vi "FF_TInial_pel.vi"() -> (0 "xyz_o":dbl[][](array[numeric]), 3 "Array":T1[](array[typedef]))   [LabVIEW 2017]
uses:
  typeDef/AnkleTraj.ctl
  <vilib>/Analysis/baseanly.llb/Real Dot Product.vi
  <vilib>/imath/engines/lvmath2/RunTimeEngine/Managers/WorkSpace/UID Generator.vi
  <vilib>/imath/engines/lvmath2/RunTimeEngine/RunTimeType/NIMS_RunTimeType_From StrictType (excl LVString).vi
  <instcachedir>/0/NIMS_RunTimeType_From StrictType (excl LVString)_1019F277F0A747EDBCA0F6C52CA54500.lvgen/NIMS_RunTimeType_From StrictType (excl LVString)_1019F277F0A747EDBCA0F6C52CA54500_000.vi
  <vilib>/imath/engines/lvmath2/RunTimeEngine/LocalVariableDefStatement/MC_LocalVariableDefStatement_Display.vi
  <vilib>/imath/engines/lvmath2/RunTimeEngine/RangeToken/NIMS_Range_R2 - Integer.vi
  <instcachedir>/0/NIMS_Range_R2 - Integer_B2C3C6B11D0E4F789E1772ACB483EB02.lvgen/NIMS_Range_R2 - Integer_B2C3C6B11D0E4F789E1772ACB483EB02_000.vi
  <vilib>/imath/engines/lvmath2/RunTimeEngine/CommandStatement/MC_CommandStatement_break.vi
  <vilib>/imath/engines/lvmath2/RunTimeEngine/VariableToken/NIMS_VariableToken_CondDefinedDefinedByReplace.vi
  <instcachedir>/0/NIMS_VariableToken_CondDefinedDefinedByReplace_D162CFFC24174562A9FEA619A91E1A56.lvgen/NIMS_VariableToken_CondDefinedDefinedByReplace_D162CFFC24174562A9FEA619A91E1A56_002.vi
  <vilib>/imath/engines/lvmath2/RunTimeEngine/IndexReplace/NIMS V(S)=S.vi
  <instcachedir>/0/NIMS V(S)=S_3F4D177D41884A9C969E5FA0B22E4B28.lvgen/NIMS V(S)=S_3F4D177D41884A9C969E5FA0B22E4B28_000.vi
  <vilib>/imathl/engines/lvmath/Functions/Error Handling/Create Error.vi
  <vilib>/imath/engines/lvmath2/RunTimeEngine/VariableToken/NIMS_VariableToken_CondDefined.vi
  <instcachedir>/0/NIMS_VariableToken_CondDefined_6E7F1EE7F80E48298C84CF05BD736261.lvgen/NIMS_VariableToken_CondDefined_6E7F1EE7F80E48298C84CF05BD736261_003.vi
  <vilib>/imath/engines/lvmath2/RunTimeEngine/BuiltInFunctions/transpose/NIMS_transpose(GV).vi
  <instcachedir>/0/NIMS_transpose(GV)_1D76875BF542458FA31D2D0CC3E998C0.lvgen/NIMS_transpose(GV)_1D76875BF542458FA31D2D0CC3E998C0_000.vi
  <vilib>/imath/engines/lvmath2/RunTimeEngine/IndexReplace/NIMS M($,S)=V.vi
  <instcachedir>/0/NIMS M($,S)=V_A7D5EE67177749758173A2B7AA759022.lvgen/NIMS M($,S)=V_A7D5EE67177749758173A2B7AA759022_001.vi
  <vilib>/imath/engines/lvmath2/RunTimeEngine/ErrorHandling/NIMS_Create Error From Enums.vi
  <vilib>/imath/engines/lvmath2/RunTimeEngine/Managers/SymbolTable/Clear UID.vi
  <vilib>/imath/engines/lvmath2/RunTimeEngine/NodeEndStatement/NIMS_NodeEndStatement_Output.vi
  <instcachedir>/0/NIMS_NodeEndStatement_Output_53EC0D466D134D7ABD903AC30B43404B.lvgen/NIMS_NodeEndStatement_Output_53EC0D466D134D7ABD903AC30B43404B_002.vi
  <vilib>/imath/engines/lvmath2/RunTimeEngine/ErrorHandling/NIMS_Finalize Error.vi
  <vilib>/Analysis/NI_AALBase.lvlib
  <vilib>/imath/engines/lvmath2/RunTimeEngine/Managers/SymbolTable/NIMS_WorkSpace.lvlib
panel:
  out "Array 2":T1[](array[typedef])
  out "Radius":i16
  out "initialized array":dbl[](array[numeric])
  out "pos":dbl[][](array[numeric])
  out "deleted portion 2":dbl[](array[numeric])
  out "all rows":dbl[][](array[numeric]) format="%0.3f"
  out "x_o":dbl[](array[numeric])
  out "array w/ subset deleted":dbl[][](array[numeric])
  in  "AnkleTraj":T1
  # "This is the input array for the force field circle"
  # "This is the array transposed"
  # "This is the output array"
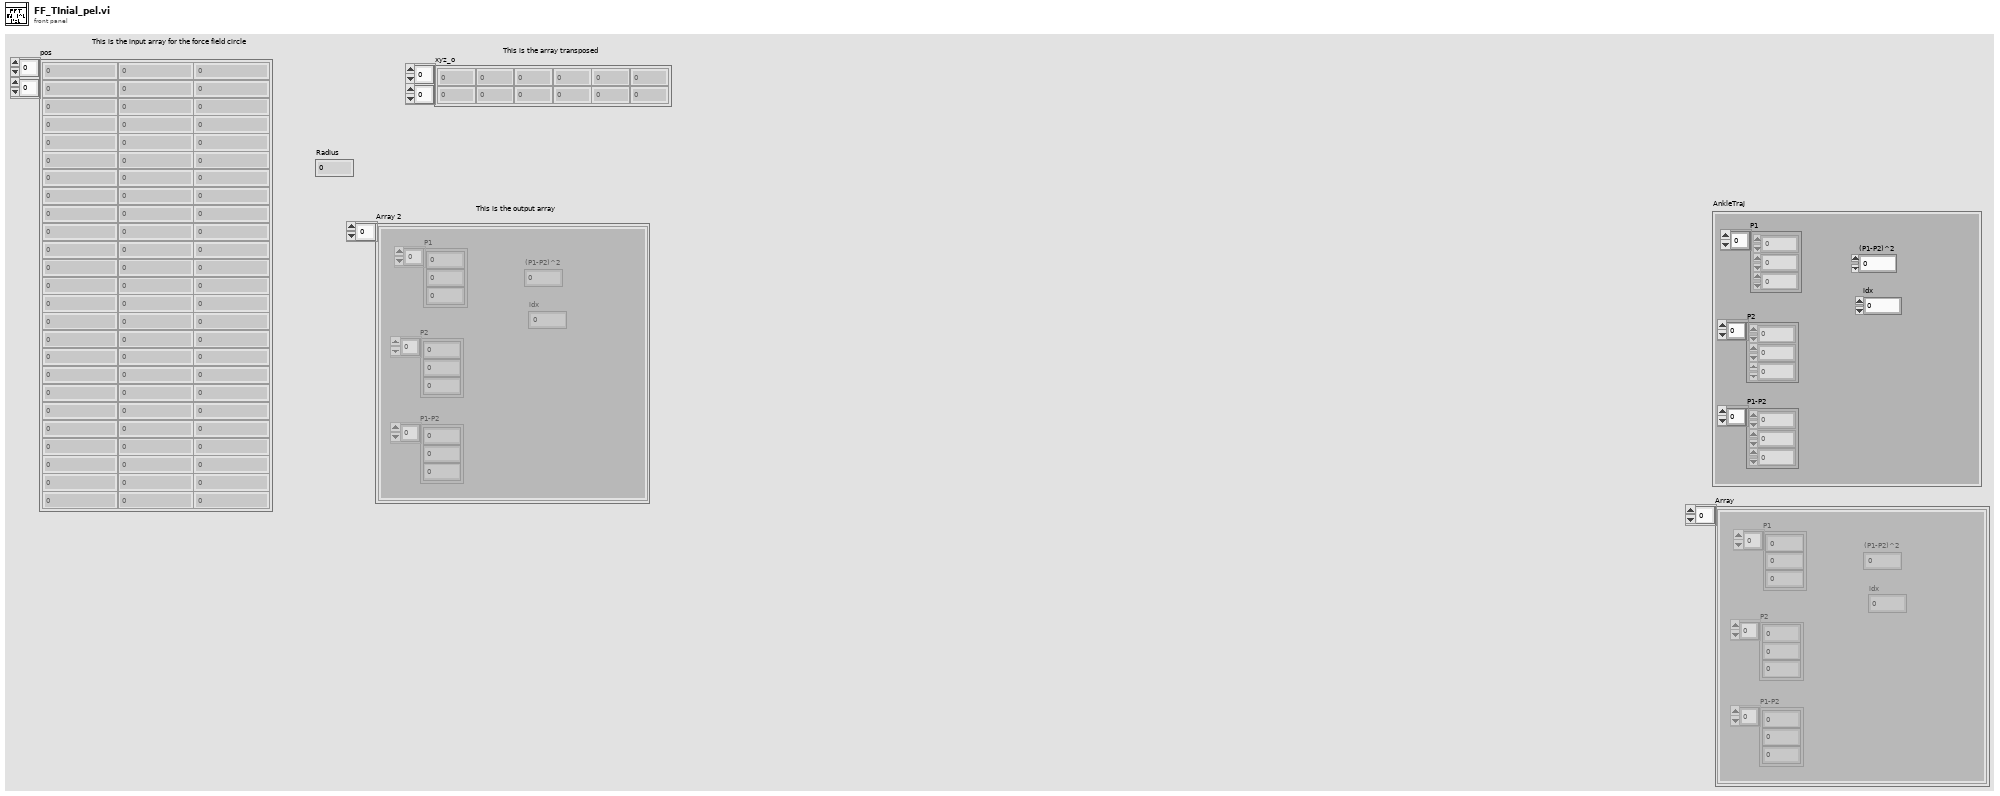
[diagram p1: front panel]
types:
  T1 = typedef "AnkleTraj.ctl" = cluster{"P1":dbl[], "P2":dbl[], "P1-P2":dbl[], "(P1-P2)^2":dbl, "idx":i32}
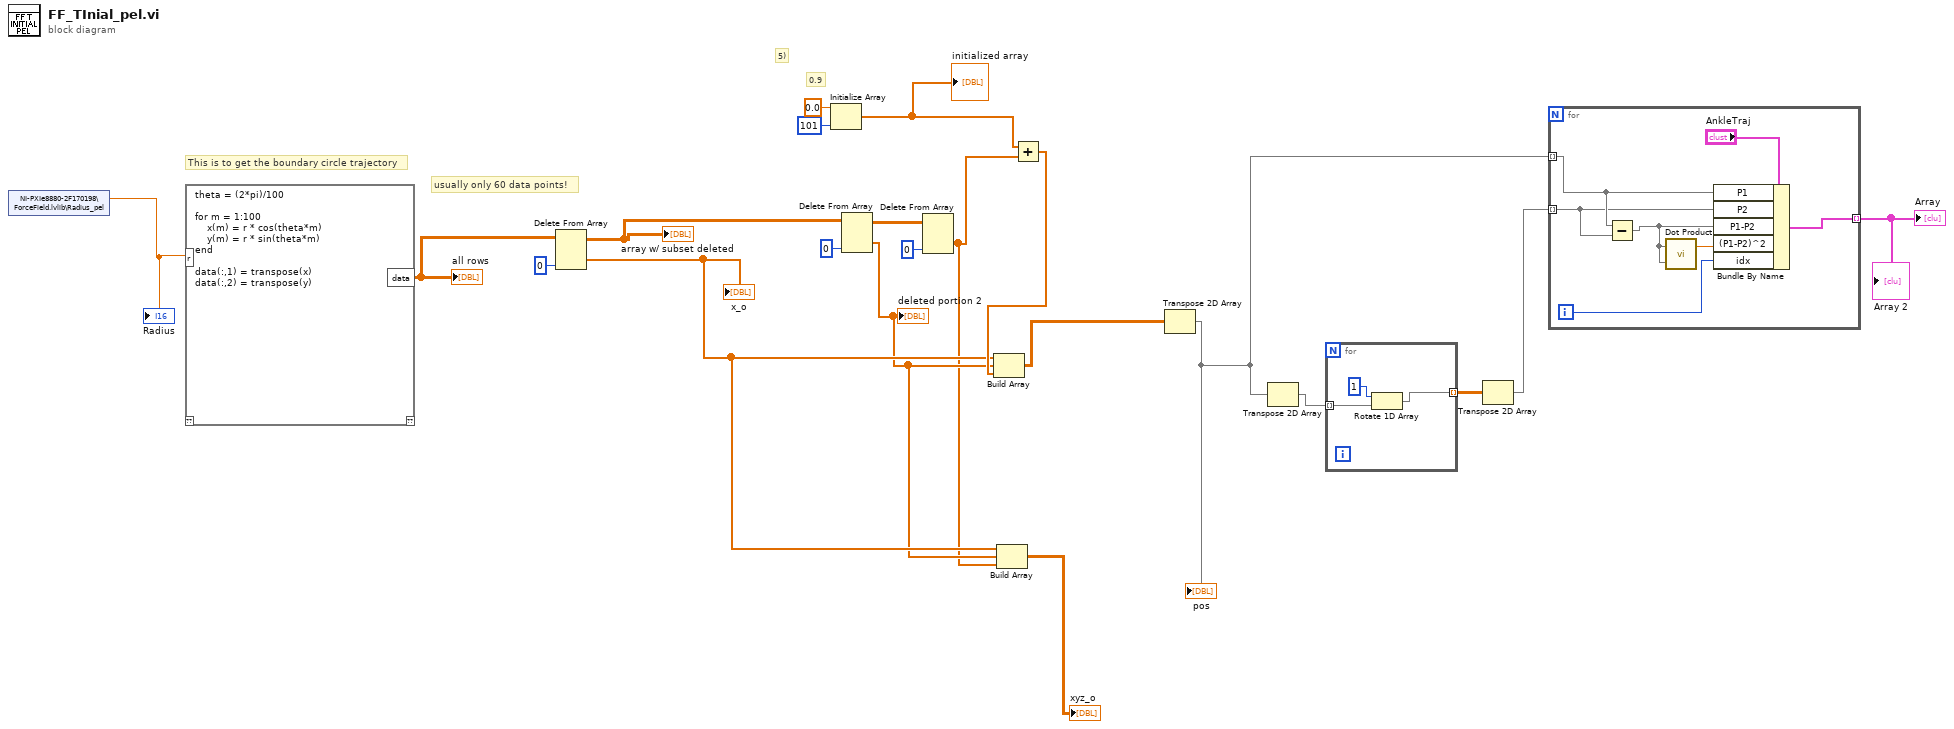
[diagram p0: block diagram]
diagram:
  # "usually only 60 data points!"
  # "5)"
  # "0.9"
  # "This is to get the boundary circle trajectory"
  n1 = shared-variable "NI-PXIe8880-2F170198\\ForceField.lvlib\\Radius_pel"() -> (w1:dbl)  [unwired: 1 in, 1 out]
  "Radius" <- w1
  n2 = mathscript code="theta = (2*pi)/100\n\nfor m = 1:100\n    x(m) = r * cos(theta*m)\n    y(m) = r * sin(theta*m)\nend\n\ndata(:,1) = transpose(x)\ndata(:,2) = transpose(y)"("r"=w1) -> ("data"=w2:dbl[][])  [unwired: 1 in, 1 out]
  "all rows" <- w2
  n3 = Delete From Array(array=w2, index (col)=0 ("disabled index (col)")) -> (deleted portion=w6:dbl[], array with subset deleted=w15:dbl[][])  [unwired: 2 in]
  "array w/ subset deleted" <- w15
  "x_o" <- w6
  n4 = Initialize Array(0.0 ("element"), 101 ("dimension size")) -> (w8:dbl[])
  "initialized array" <- w8
  n5 = Delete From Array(array=w15, index (col)=0) -> (deleted portion=w5:dbl[], array with subset deleted=w14:dbl[][])  [unwired: 2 in]
  "deleted portion 2" <- w5
  n6 = Delete From Array(array=w14, index (col)=0 ("disabled index (col)")) -> (deleted portion=w4:dbl[])  [unwired: 2 in, 1 out]
  n7 = Build Array(w6, w5, w4) -> (→"xyz_o":dbl[][])
  n8 = Add(x=w8, y=w4) -> (x+y=w7:dbl[])
  n9 = Build Array(w6, w5, w7) -> (w11:dbl[][])
  n10 = Transpose 2D Array(2D array=w11) -> (transposed array=w12:dbl[][])
  "pos" <- w12
  n11 = Transpose 2D Array(2D array=w12) -> (transposed array=w21:dbl[][])
  n12 = for {
    tunnel: w21 -> [w24] mode=indexing
    tunnel: [w23] -> w20 mode=indexing
    n13 = Rotate 1D Array(1:w24, 2:1 ("n")) -> (0:w23:dbl[])
  }
  n14 = Transpose 2D Array(2D array=w20) -> (transposed array=w19:dbl[][])
  n15 = for {
    tunnel: w12 -> [w30] mode=indexing
    tunnel: w19 -> [w29] mode=indexing
    tunnel: [w26] -> w18 mode=indexing
    i -> [w25]
    n16 = Subtract(x=w30, y=w29) -> (x-y=w27:dbl[])
    n17 = call-poly <vilib>:"Dot Product.vi"("Y Vector"=w27, "X Vector"=w27) -> ("X * Y"=w28:dbl)  [unwired: 1 out]
    n18 = Bundle By Name(cluster="AnkleTraj", "P1"=w30, "P2"=w29, "P1-P2"=w27, "(P1-P2)^2"=w28, "idx"=w25) -> (w26:T1)
  }
  "Array" <- w18
  "Array 2" <- w18
